vi "lsl get fullinfo.vi"(8 "error in (no error)":errorcluster, 9 "ec":i32, 10 "timeout":dbl, 11 "in":cluster{}) -> (0 "error out":errorcluster, 1 "ec out":i32, 2 "function return":u32, 3 "in out":cluster{})   [LabVIEW 2018, in "liblsl-LabVIEW.lvlib"]
doc: "extern LIBLSL_C_API lsl_streaminfo lsl_get_fullinfo(lsl_inlet in, double timeout, int32_t *ec);"
uses:
  <userlib>/liblsl-LabVIEW/liblsl-LabVIEW.lvlib
  <userlib>/liblsl-LabVIEW/liblsl64.dll
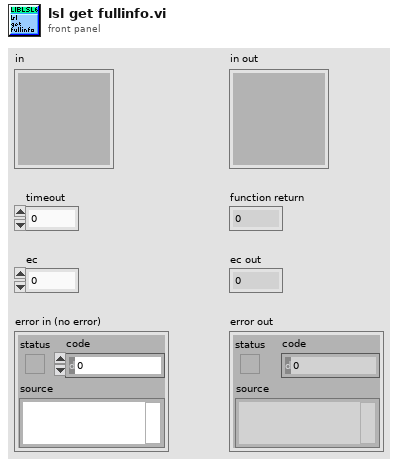
[diagram p1: front panel]
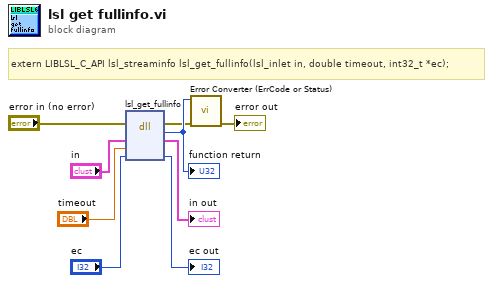
[diagram p0: block diagram]
diagram:
  # "extern LIBLSL_C_API lsl_streaminfo lsl_get_fullinfo(lsl_inlet in, double timeout, int32_t *ec);"
  n1 = dll-call lib="C:/Program Files/National Instruments/LabVIEW 2018/user.lib/liblsl-LabVIEW/liblsl64.*" fn="lsl_get_fullinfo"(error in="error in (no error)", "in"="in", "timeout"="timeout", "ec"="ec") -> (error out=w2:errorcluster, w9:u32, "in"=→"in out":cluster{}, "ec"=→"ec out":i32)  [unwired: 3 in, 1 out]
  "function return" <- w9
  n2 = call <userlib>:"Error Converter (ErrCode or Status).vi"("error in (no error)"=w2, "error code"=w9) -> ("error out"=→"error out":errorcluster)  [unwired: 9 in]
